vi "Fdx Close Rx UDP Session.vi"(8 "error in (no error)":errorcluster, 10 "UdpHandle in":u32, 11 "InstrumentHandle_port in":u32) -> (0 "error out":errorcluster, 3 "InstrumentHandle_port out":u32)   [LabVIEW 2020, in "AIM664LV.lvlib"]
uses:
  AIM664LV.lvlib
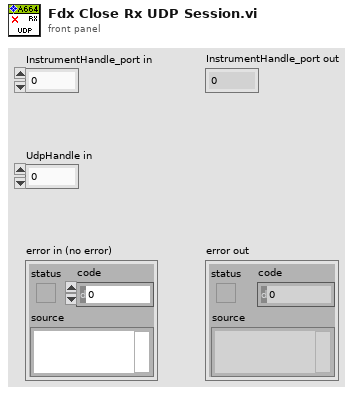
[diagram p1: front panel]
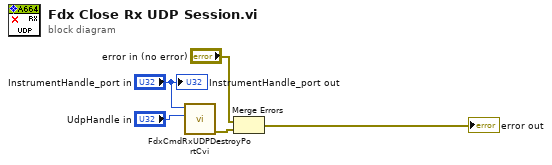
[diagram p0: block diagram]
diagram:
  n1 = call "FdxCmdRxUDPDestroyPortCvi.vi"("UdpHandle"="UdpHandle in", "InstrumentHandle_port"="InstrumentHandle_port in") -> ("error out"=w3:errorcluster)  [unwired: 8 in, 1 out]
  n2 = Merge Errors("error in (no error)", w3) -> (→"error out":errorcluster)
  "InstrumentHandle_port out" <- "InstrumentHandle_port in"
